vi "sendMessage.vi"(0 "Token":string, 5 "MsgType":T1, 7 "ChatId":i32, 9 "Text":string, 11 "error in":errorcluster, 12 "ReplyKeyboardMarkup":T2, 13 "reply_to_message_id":i32) -> (15 "error out":errorcluster)   [LabVIEW 2015]
uses:
  TypeDefs/ReplyKeyboardMarkup.ctl
  TypeDefs/SendMessageType.ctl
  TypeDefs/sendMessage.ctl
  <vilib>/httpClient/LabVIEWHTTPClient.lvlib
panel:
  out "Token":string
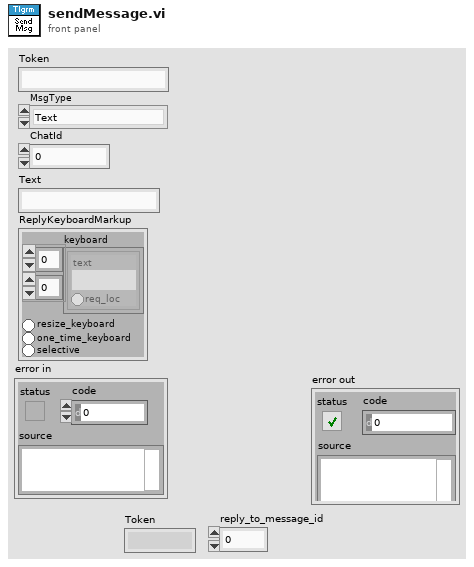
[diagram p1: front panel]
types:
  T1 = typedef "SendMessageType.ctl" = enum16{"Text", "ReplyKeyboardMarkup", "ReplyKeyboardRemove"}
  T2 = typedef "ReplyKeyboardMarkup.ctl" = cluster{"keyboard":cluster{"text":string, "req_loc":bool}[][], "resize_keyboard":bool, "one_time_keyboard":bool, "selective":bool}
  T3 = cluster{"remove_keyboard":bool, "selective":bool}
  T4 = typedef "sendMessage.ctl" = cluster{"chat_id":string, "reply_to_message_id":string, "text":string, "reply_markup":string}
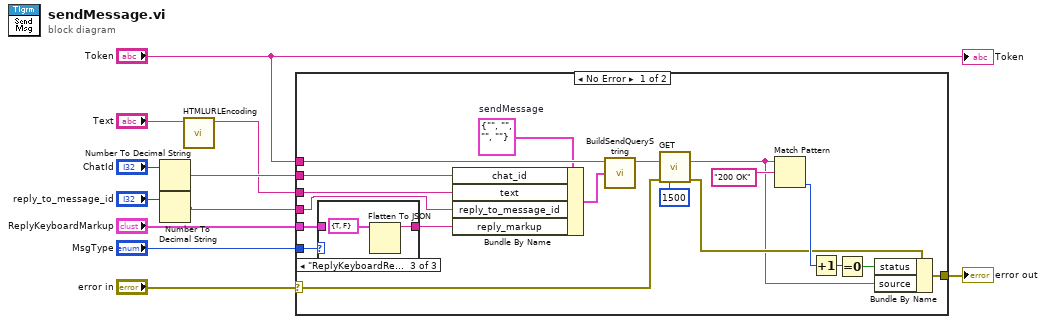
[diagram p0: block diagram]
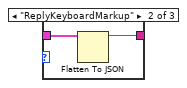
[diagram p3: hidden frame]
diagram:
  n1 = Number To Decimal String(number="ChatId") -> (decimal integer string=w5:string)  [unwired: 1 in]
  n2 = Number To Decimal String(number="reply_to_message_id") -> (decimal integer string=w3:string)  [unwired: 1 in]
  n3 = call "HTMLURLEncoding.vi"("InputString"="Text") -> ("URLEncodedString"=w2:string)  [unwired: 10 in]
  n4 = case shown="No Error" "error in" {
    selector: "error in" -> [w15 w35]
    tunnel: "Token" -> [w21 _]
    tunnel: [w25 w35] -> w11
    tunnel: "ReplyKeyboardMarkup" -> [w17 _]
    tunnel: "MsgType" -> [w16 _]
    tunnel: w5 -> [w14 _]
    tunnel: w2 -> [w13 _]
    tunnel: w3 -> [w12 _]
    frame No Error {
      w20 = T4 {"chat_id"="", "reply_to_message_id"="", "text"="", "reply_markup"=""}  # sendMessage
      n5 = case shown="\"ReplyKeyboardRemove\"" w16 {
        tunnel: [_ w32 w34] -> w18
        tunnel: w17 -> [_ w31 _]
        frame Default {
        }
        frame "ReplyKeyboardMarkup" {
          n6 = Flatten To JSON(anything=w31) -> (JSON string=w32:string)  [unwired: 2 in, 1 out]
        }
        frame "ReplyKeyboardRemove" {
          n7 = Flatten To JSON(anything=T3 {"remove_keyboard"=TRUE, "selective"=FALSE} ("ReplyKeyboardRemove")) -> (JSON string=w34:string)  [unwired: 2 in, 1 out]
        }
      }
      n8 = Bundle By Name(cluster=w20, "chat_id"=w14, "text"=w13, "reply_to_message_id"=w12, "reply_markup"=w18) -> (w19:T4)
      n9 = call "BuildSendQueryString.vi"("sendMessage"=w19, "Token"=w21) -> ("QueryStringOut"=w22:string)  [unwired: 9 in]
      n10 = call <vilib>:"GET.vi"("url"=w22, "error in (no error)"=w15, "timeout (10000)"=1500) -> ("headers"=w23:string, "error out"=w26:errorcluster)  [unwired: 9 in, 2 out]
      n11 = Match Pattern(string=w23, regular expression="200 OK") -> (offset past match=w28:i32)  [unwired: 1 in, 3 out]
      n12 = Increment(x=w28) -> (x+1=w27:i32)
      n13 = Equal To 0?(x=w27) -> (x = 0?=w24:bool)
      n14 = Bundle By Name(cluster=w26, "status"=w24, "source"=w23) -> (w25:errorcluster)
    }
    frame Error {
    }
  }
  "error out" <- w11
  "Token" <- "Token"
